vi "Xml_Save_As_File.vi"(8 "error in (no error)":errorcluster, 10 "EXPERT Path Selector":T7=enum."XML Saved", 11 "Variant":variant) -> (0 "error out":errorcluster)   [LabVIEW 2017]
uses:
  controls/EXPERT_Path_Selector.ctl
  controls/QMH_UI_Cluster.ctl
  controls/QMH_UI_References.ctl
  controls/QMH_UI_Report.ctl
  controls/QMH_UI_Command.ctl
  controls/QMH_ICR_Command.ctl
  controls/QMH_Status.ctl
panel:
  in  "QMH UI Cluster":T1
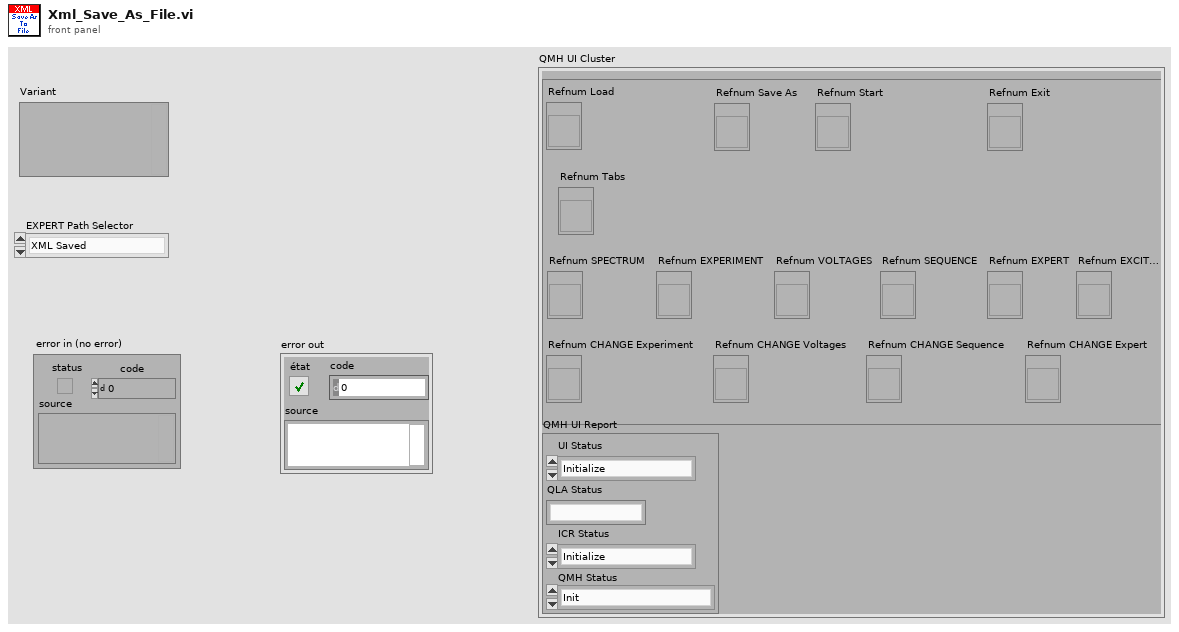
[diagram p1: front panel]
types:
  T1 = typedef "QMH_UI_Cluster.ctl" = cluster{"QMH UI References":T2, "QMH UI Report":T3}
  T2 = typedef "QMH_UI_References.ctl" = cluster{"Refnum Load":refnum<vi>, "Refnum Save As":refnum<vi>, "Refnum Start":refnum<vi>, "Refnum Exit":refnum<vi>, "Refnum Tabs":refnum<vi>, "Refnum SPECTRUM":refnum<vi>, "Refnum EXPERIMENT":refnum<vi>, "Refnum VOLTAGES":refnum<vi>, "Refnum SEQUENCE":refnum<vi>, "Refnum EXPERT":refnum<vi>, "Refnum EXCIT Table":refnum<vi>, "Refnum TIMING Table":refnum<vi>, "Refnum CHANGE Experiment":refnum<vi>, "Refnum CHANGE Voltages":refnum<vi>, "Refnum CHANGE Sequence":refnum<vi>, "Refnum CHANGE Expert":refnum<vi>, "Refnum CHANGE Scientist":refnum<vi>}
  T3 = typedef "QMH_UI_Report.ctl" = cluster{"UI Status":T4, "QLA Status":string, "ICR Status":T5, "QMH Status":T6}
  T4 = typedef "QMH_UI_Command.ctl" = enum16{"Initialize", "UI Load", "UI Save", "UI Save As", "UI Change Experiment", "UI Change Voltages", "UI Change Sequence", "UI Change Expert", "UI Change Scientist", "Ready to Start", "UI Start", "Waiting for ICR", "UI Exit", "Update Report", "Update ICR Report"}
  T5 = typedef "QMH_ICR_Command.ctl" = enum16{"Initialize", "Sequence Setup", "ICR Start", "ICR Stop", "Hardware Setup", "Next Accumulation", "Waiting for Trigger", "Sequence Started", "Sequence Finished", "Writing Data", "Hardware Reset", "Exit"}
  T6 = typedef "QMH_Status.ctl" = enum16{"Init", "Loading", "Setup", "Ready to Start", "Started", "Idle"}
  T7 = typedef "EXPERT_Path_Selector.ctl" = enum16{"Application", "Resources", "Data", "XML", "XML Saved", "Load Directory"}
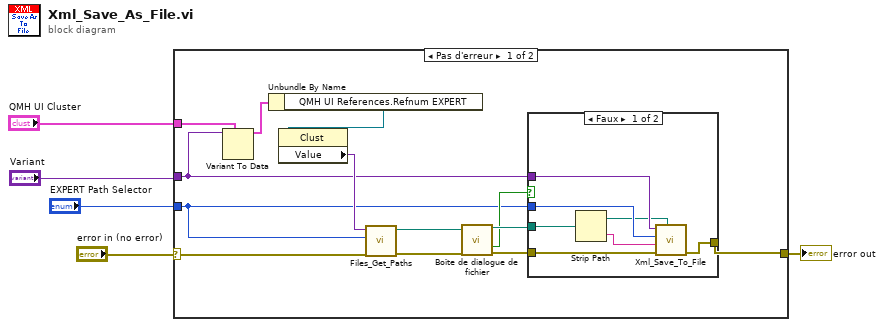
[diagram p0: block diagram]
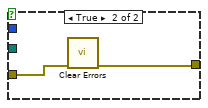
[diagram p2: hidden frame]
diagram:
  n1 = case shown="Pas d'erreur" "error in (no error)" {
    selector: "error in (no error)" -> [w14 w28]
    tunnel: "Variant" -> [w9 _]
    tunnel: [w15 w28] -> w4
    tunnel: "EXPERT Path Selector" -> [w7 _]
    tunnel: "QMH UI Cluster" -> [w6 _]
    frame No Error {
      n2 = Variant To Data(type=w6, Variant=w9) -> (data=w12:T1)  [unwired: 1 in, 1 out]
      n3 = Unbundle By Name(w12) -> ("QMH UI References.Refnum EXPERT"=w11:refnum<vi>)
      n4 = property class="Clust"(reference=w11) -> ("Value"=w10:variant)  [unwired: 1 in, 2 out]
      n5 = call "Files_Get_Paths.vi"("error in (no error)"=w14, "EXPERT Path Selector"=w7, "Variant"=w10) -> ("error out"=w8:errorcluster, "Path"=w13:path)  [unwired: 7 in]
      n6 = call "Boîte de dialogue de fichier"("start path"=w13, "error in"=w8) -> ("selected path"=w18:path, "cancelled"=w16:bool, "error out"=w17:errorcluster)  [unwired: 10 in, 1 out]
      n7 = case shown="Faux" w16 {
        tunnel: w18 -> [w23 _]
        tunnel: w17 -> [w24 w27]
        tunnel: [w25 w26] -> w15
        tunnel: w9 -> [w21 _]
        tunnel: w7 -> [w20 _]
        frame False {
          n8 = Strip Path(path=w23) -> (stripped path=w19:path, name=w22:string)
          n9 = call "Xml_Save_To_File.vi"("Custom Path"=w19, "error in (no error)"=w24, "Filename"=w22, "EXPERT Path Selector"=w20, "Variant"=w21) -> ("error out"=w25:errorcluster)  [unwired: 6 in]
        }
        frame True {
          n10 = call <vilib>:"Clear Errors.vi"("error in (no error)"=w27) -> ("error out"=w26:errorcluster)  [unwired: 5 in, 1 out]
        }
      }
    }
    frame Error {
    }
  }
  "error out" <- w4
